vi "Init.vi"(0 "Resource Name":string, 1 "ID Query":i32(ring)=1 items=["Do Query"=1, "Skip Query"=0], 2 "Reset":i32(ring) items=["Reset Device"=1, "Don't Reset"=0], 3 "error in":errorcluster, 4 "Comm Bus":u16(ring)=2 items=["ZT_MCLASS"=2, "ZT_LAN"=4, "ZT_VISA_PCI_M"=258, "ZT_VISA_M"=514]) -> (7 "Instr Handle":i32 caption="Instrument Handle", 8 "Model Number":u32, 10 "error out":errorcluster)   [LabVIEW 2013, in "ZTScopeM.lvlib"]
doc: "Establish an instrument communication session."
uses:
  ZTScopeM.lvlib
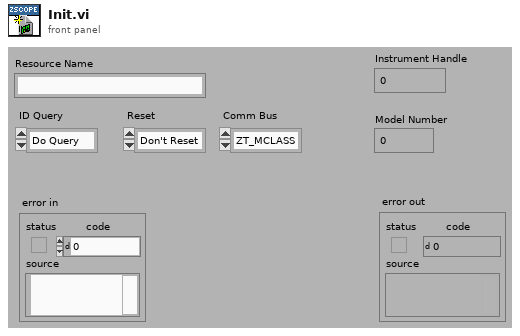
[diagram p1: front panel]
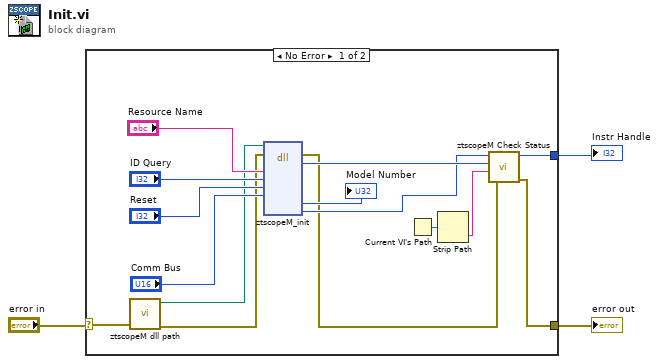
[diagram p0: block diagram]
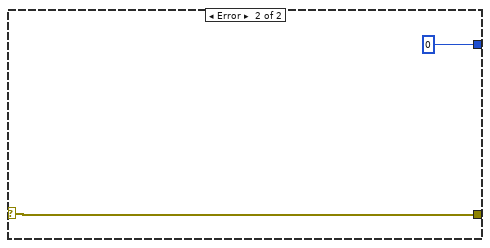
[diagram p2: hidden frame]
diagram:
  n1 = case shown="No Error" "error in" {
    selector: "error in" -> [w7 w19]
    tunnel: [w11 w19] -> w2
    tunnel: [w12 0 ("instrumentHandle")] -> w1
    frame No Error {
      n2 = call "ztscopeM dll path.vi"("error in (no error)"=w7) -> ("error out"=w5:errorcluster, "<instrument>.dll path"=w6:path)  [unwired: 9 in]
      n3 = dll-call lib="C:/Program Files (x86)/National Instruments/LabVIEW 2013/instr.lib/ztscopem/ztscopeM.dll" fn="ztscopeM_init"(path in=w6, error in=w5, "resourceName"="Resource Name", "IDQuery"="ID Query", "reset"="Reset", "comm_bus"="Comm Bus") -> (error out=w4:errorcluster, w15:i32, "model_number"=→"Model Number":u32, "instrumentHandle"=w10:i32)  [unwired: 7 in, 1 out]
      n4 = Current VI's Path() -> (path=w14:path)
      n5 = Strip Path(path=w14) -> (name=w13:string)  [unwired: 1 out]
      n6 = call "ztscopeM Check Status.vi"("error in"=w4, "name of VI"=w13, "status (return code)"=w15, "instrument handle in"=w10) -> ("error out"=w11:errorcluster, "instrument handle out"=w12:i32)  [unwired: 2 in]
    }
    frame Error {
    }
  }
  "Instr Handle" <- w1
  "error out" <- w2
